vi "Divide.vi"(1 "x":sgl, 2 "y":sgl, 4 "Divider1":refnum<class "Divider1.lvclass">) -> (6 "x/y":sgl)   [LabVIEW 2017, in "Divider1.lvclass"]
uses:
  Divider1.lvclass
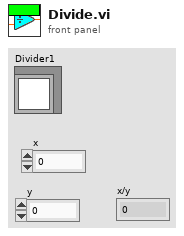
[diagram p1: front panel]
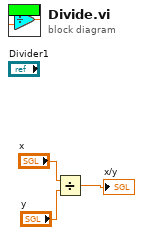
[diagram p0: block diagram]
diagram:
  n1 = Divide(x="x", y="y") -> (x/y=→"x/y":sgl)
